vi "Init.vi"(8 "error in (no error)":errorcluster, 11 "FIFO Reader in":refnum<class "FIFO Reader.lvclass">) -> (0 "error out":errorcluster, 3 "FIFO Reader out":refnum<class "FIFO Reader.lvclass">)   [LabVIEW 2024, in "RIO Streamer.lvlib" / "FIFO Reader.lvclass"]
uses:
  FIFO Reader.lvclass
  SubVI/NiVeriStandFpgaDmaXml.ctl
  FIFO Reader.lvclass/FIFO Reader.ctl
panel:
  out "value":T1
  in  "Device address":string
  in  "Path":path=path "C:/_git/FlexLogger-RioStreamer/fpga/R Series Example.fpgaconfig"
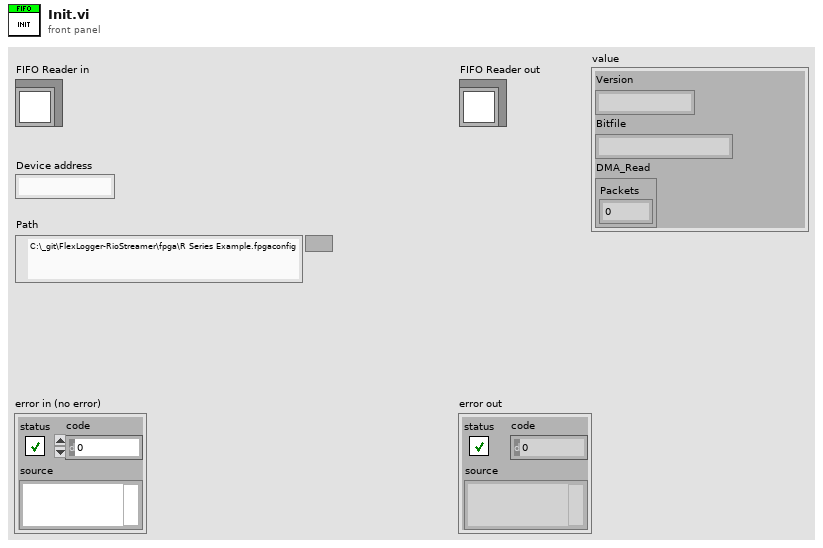
[diagram p1: front panel]
types:
  T1 = typedef "RIO Streamer.lvlib/FIFO Reader.lvclass/NiVeriStandFpgaDmaXml.ctl" = cluster{"Version":string, "Bitfile":string, "DMA_Read":cluster{"Packets":dbl}}
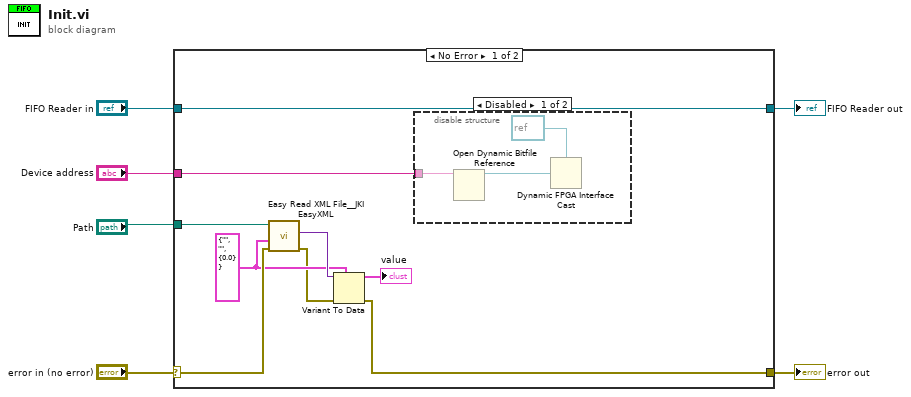
[diagram p0: block diagram]
diagram:
  n1 = case shown="No Error" "error in (no error)" {
    selector: "error in (no error)" -> [w12 w20]
    tunnel: [w7 w20] -> w6
    tunnel: [w15 w19] -> w4
    tunnel: "FIFO Reader in" -> [w15 w19]
    tunnel: "Device address" -> [w14 _]
    tunnel: "Path" -> [w13 _]
    frame No Error {
      w10 = T1 {"Version"="", "Bitfile"="", "DMA_Read"={"Packets"=0.0}}
      n2 = call <vilib>:"Easy Read XML File__JKI EasyXML.vi"("error in (no error)"=w12, "LabVIEW Data (Type)"=w10, "XML File Path"=w13) -> ("error out"=w9:errorcluster, "LabVIEW Data"=w11:variant)  [unwired: 6 in, 1 out]
      n3 = Variant To Data(error in=w9, type=w10, Variant=w11) -> (data=→"value":T1, error out=w7:errorcluster)
      n4 = disable-structure shown="Disabled" {
        disable-tunnel: w14 -> [w17 _]
        frame Disabled {
          n5 = Open Dynamic Bitfile Reference(0:w17) -> (5:w18:refnum<k20>)  [unwired: 4 in, 1 out]
          n6 = Dynamic FPGA Interface Cast(Session In=refnum<k20> refnum ("Type"), Type=w18) -> ()  [unwired: 1 out]
        }
        frame Enabled {
        }
      }
    }
    frame Error {
    }
  }
  "error out" <- w6
  "FIFO Reader out" <- w4
